vi "SignalPanelDev.vi"(8 "error in (no error)":errorcluster caption="entrée d'erreur (pas d'erreur)", 10 "Message":cluster{"Message":string, "Data":variant, i32}, 11 "Experiment en entrée":refnum<class "Experiment.lvclass"> caption="DNL_LabVIEW Object in") -> (0 "error out":errorcluster caption="sortie d'erreur", 3 "Experiment en sortie":refnum<class "Experiment.lvclass"> caption="DNL_LabVIEW Object out")   [LabVIEW 2019, in "Experiment.lvclass"]
uses:
  Experiment.lvclass
  Experiment.lvclass/Experiment.ctl
  DevicesClass/BaseDevice/Accessor/GetClassEvent.vi
  DevicesClass/BaseDevice/Accessor/GetClassQueue.vi
  DevicesClass/BaseDevice/BaseDevice.lvclass
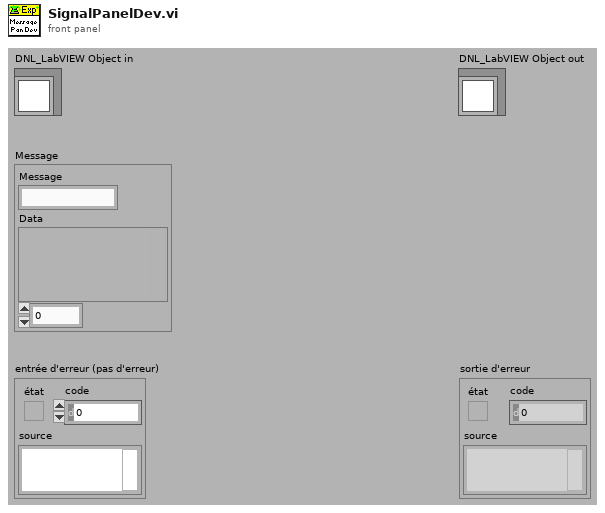
[diagram p1: front panel]
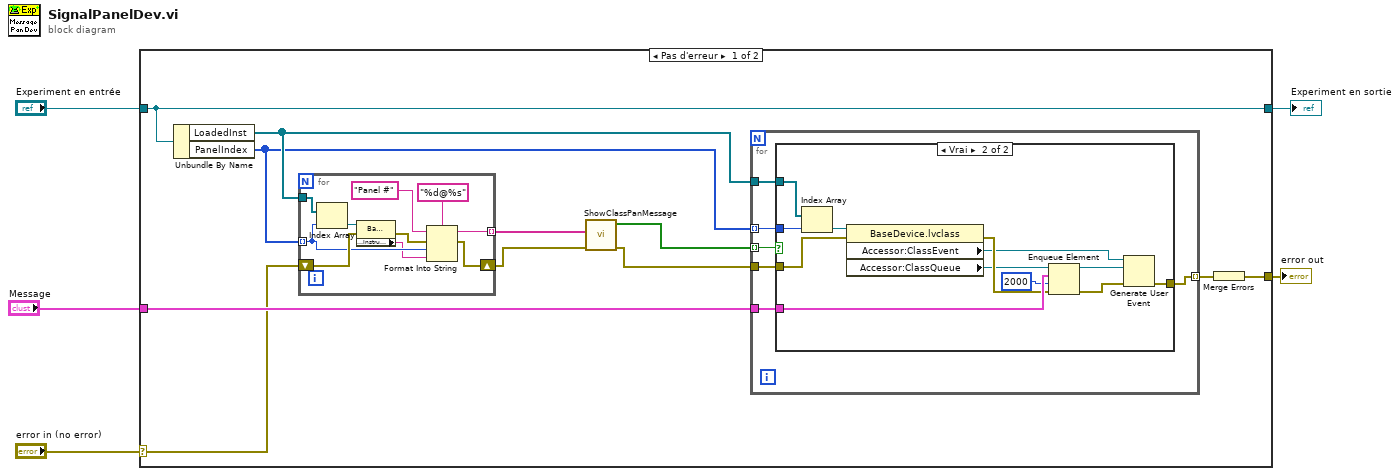
[diagram p0: block diagram]
diagram:
  n1 = case shown="Pas d'erreur" "error in (no error)" {
    selector: "error in (no error)" -> [w10 w47]
    tunnel: [w14 w47] -> w4
    tunnel: [w16 w46] -> w2
    tunnel: "Experiment en entrée" -> [w16 w46]
    tunnel: "Message" -> [w13 _]
    frame No Error {
      n2 = Unbundle By Name(w16) -> ("LoadedInst"=w12:refnum<class "BaseDevice.lvclass">[], "PanelIndex"=w11:i32[])
      n3 = for {
        tunnel: w12 -> [w25]
        tunnel: w11 -> [w19] mode=indexing
        shift-right: [w22] -> w8
        shift-left: w10 -> [w23]
        tunnel: [w17] -> w9 mode=indexing
        n4 = Index Array(array=w25, index=w19) -> (element=w26:refnum<class "BaseDevice.lvclass">)
        n5 = property class="BaseDevice.lvclass"(reference=w26, error in=w23) -> (error out=w24:errorcluster, "Accessor:InstrumentName"=w18:string)  [unwired: 1 out]
        n6 = Format Into String(format string="%d@%s" ("chaîne de format"), initial string="Panel #" ("chaîne initiale"), error in=w24, w19, w18) -> (resulting string=w17:string, error out=w22:errorcluster)
      }
      n7 = call "ShowClassPanMessage.vi"("ErrorIn(NoErr)"=w8, "Tableau"=w9) -> ("ErrorOut(NoErr)"=w7:errorcluster, "Show"=w6:bool[])  [unwired: 8 in]
      n8 = for {
        tunnel: w12 -> [w32]
        tunnel: w11 -> [w28] mode=indexing
        tunnel: w7 -> [w31]
        tunnel: [w30] -> w15 mode=indexing
        tunnel: w13 -> [w29]
        tunnel: w6 -> [w27] mode=indexing
        n9 = case shown="Vrai" w27 {
          tunnel: w32 -> [_ w45]
          tunnel: w31 -> [w33 w44]
          tunnel: [w33 w43] -> w30
          tunnel: w29 -> [_ w42]
          tunnel: w28 -> [_ w35]
          frame False {
          }
          frame True {
            n10 = Index Array(array=w45, index=w35) -> (element=w41:refnum<class "BaseDevice.lvclass">)
            n11 = property class="BaseDevice.lvclass"(reference=w41, error in=w44) -> (error out=w38:errorcluster, "Accessor:ClassEvent"=w37:refnum<user-event>, "Accessor:ClassQueue"=w36:refnum<queue>)  [unwired: 1 out]
            n12 = Enqueue Element(queue=w36, element=w42, timeout in ms (-1)=2000 ("timeout en ms (-1)"), error in (no error)=w38) -> (queue out=w40:refnum<queue>, error out=w39:errorcluster)  [unwired: 1 out]
            n13 = Generate User Event(user event=w37, event data cluster=w40, error in=w39) -> (error out=w43:errorcluster)  [unwired: 1 in, 1 out]
          }
        }
      }
      n14 = Merge Errors(w15) -> (w14:errorcluster)
    }
    frame Error {
    }
  }
  "error out" <- w4
  "Experiment en sortie" <- w2
